vi "Read Encoder Position.vi"(11 "EnccoderConverter in":refnum<class "EncoderConverter.lvclass">) -> (2 "EnccoderConverter Position":dbl[unit], 3 "EnccoderConverter out":refnum<class "EncoderConverter.lvclass">)   [LabVIEW 2015, in "EncoderConverter.lvlib" / "EncoderConverter.lvclass"]
uses:
  <userlib>/Common/Devices/EncoderConverter/EncoderConverter/EncoderConverter.lvclass
  <userlib>/Common/Devices/EncoderConverter/EncoderConverter/EncoderConverter.lvclass/EncoderConverter.ctl
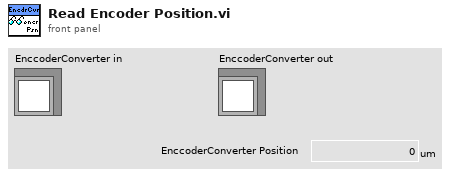
[diagram p1: front panel]
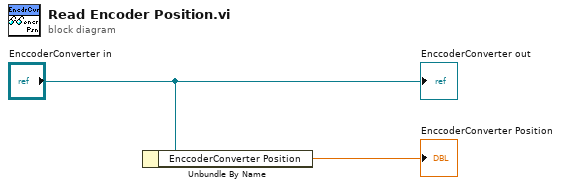
[diagram p0: block diagram]
diagram:
  n1 = Unbundle By Name("EnccoderConverter in") -> ("EnccoderConverter Position"=→"EnccoderConverter Position":dbl[unit])
  "EnccoderConverter out" <- "EnccoderConverter in"
